vi "moyenne.vi"(8 "Y":i32(knob)=1 min=-10 max=10 scale=-20.0..20.0, 11 "X":i32(knob)=1 min=-10 max=10 scale=-20.0..20.0) -> (3 "Moyenne":ext)   [LabVIEW 2025]
doc: "Fait la moyenne entre x et y"
panel:
  out "Positif?":bool
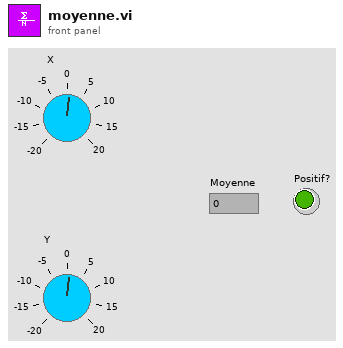
[diagram p1: front panel]
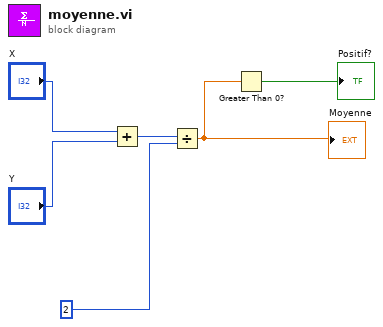
[diagram p0: block diagram]
diagram:
  n1 = Add(x="X", y="Y") -> (x+y=w6:i32)
  n2 = Divide(x=w6, y=2) -> (x/y=w1:dbl)
  "Moyenne" <- w1
  n3 = Greater Than 0?(x=w1) -> (x > 0?=→"Positif?":bool)
